vi "SIAM-7xRollingShutter.vi"() -> ()   [LabVIEW 2011]
uses:
  SIAM_command.ctl
panel:
  in  "Wob/µm":dbl=62.993226
  in  "Grid µm":dbl=29.0
  out "set Camera Exposure [µs]":dbl=743.175
  in  "PhaseImages":u16=7
  in  "GalvoX-Blanking":dbl
  in  "NoOfImages":u16=35
  out "µmShift":dbl=10.96096971726759 format="%#_8g"
  in  "Camera-Lines":u32=1082
  in  "Turn_ticks":u32=120
  in  "SM_ticks":u32=116
  in  "Trigger_ticks":u32=100
  in  "Mask_tpos":dbl=45853.0
  in  "LineTime-µs":dbl=27.525
  in  "RollingShutter height":u16=27
  in  "galvox/pixel":dbl=7.407
  in  "galvox-Line1080":dbl=-12220.0
  out "SIAMScript":T2(array[cluster])=[{"Delay 10µs"=50, "command"=1612709953, "P0"=0, "P1"=-269103235, "P2"=0, "P3"=0, "P4"=0, "P5-ticket"=0}, {"Delay 10µs"=0, "command"=1611661377, "P0"=0, "P1"=0, "P2"=0, "P3"=0, "P4"=0, "P5-ticket"=0}, {"Delay 10µs"=120, "command"=1612709921, "P0"=0, "P1"=0, "P2"=-2821727, "P3"=0, "P4"=0, "P5-ticket"=0}, {"Delay 10µs"=113, "command"=3506438145, "P0"=1, "P1"=1, "P2"=0, "P3"=0, "P4"=0, "P5-ticket"=0}, {"Delay 10µs"=100, "command"=3506438145, "P0"=1, "P1"=0, "P2"=0, "P3"=0, "P4"=0, "P5-ticket"=0}, {"Delay 10µs"=2856, "command"=1612709921, "P0"=0, "P1"=0, "P2"=0, "P3"=0, "P4"=0, "P5-ticket"=0}, {"Delay 10µs"=50, "command"=1612709953, "P0"=0, "P1"=-269103235, "P2"=0, "P3"=0, "P4"=0, "P5-ticket"=0}, {"Delay 10µs"=0, "command"=1611661377, "P0"=0, "P1"=45250435, "P2"=0, "P3"=0, "P4"=0, "P5-ticket"=0}, {"Delay 10µs"=120, "command"=1612709921, "P0"=0, "P1"=0, "P2"=-2821727, "P3"=0, "P4"=0, "P5-ticket"=0}, {"Delay 10µs"=113, "command"=3506438145, "P0"=1, "P1"=1, "P2"=0, "P3"=0, "P4"=0, "P5-ticket"=0}, {"Delay 10µs"=100, "command"=3506438145, "P0"=1, "P1"=0, "P2"=0, "P3"=0, "P4"=0, "P5-ticket"=0}, {"Delay 10µs"=2856, "command"=1612709921, "P0"=0, "P1"=0, "P2"=0, "P3"=0, "P4"=0, "P5-ticket"=0}, {"Delay 10µs"=50, "command"=1612709953, "P0"=0, "P1"=-269103235, "P2"=0, "P3"=0, "P4"=0, "P5-ticket"=0}, {"Delay 10µs"=0, "command"=1611661377, "P0"=0, "P1"=90500870, "P2"=0, "P3"=0, "P4"=0, "P5-ticket"=0}, {"Delay 10µs"=120, "command"=1612709921, "P0"=0, "P1"=0, "P2"=-2821727, "P3"=0, "P4"=0, "P5-ticket"=0}, {"Delay 10µs"=113, "command"=3506438145, "P0"=1, "P1"=1, "P2"=0, "P3"=0, "P4"=0, "P5-ticket"=0}, {"Delay 10µs"=100, "command"=3506438145, "P0"=1, "P1"=0, "P2"=0, "P3"=0, "P4"=0, "P5-ticket"=0}, {"Delay 10µs"=2856, "command"=1612709921, "P0"=0, "P1"=0, "P2"=0, "P3"=0, "P4"=0, "P5-ticket"=0}, {"Delay 10µs"=50, "command"=1612709953, "P0"=0, "P1"=-269103235, "P2"=0, "P3"=0, "P4"=0, "P5-ticket"=0}, {"Delay 10µs"=0, "command"=1611661377, "P0"=0, "P1"=135751305, "P2"=0, "P3"=0, "P4"=0, "P5-ticket"=0}, {"Delay 10µs"=120, "command"=1612709921, "P0"=0, "P1"=0, "P2"=-2821727, "P3"=0, "P4"=0, "P5-ticket"=0}, {"Delay 10µs"=113, "command"=3506438145, "P0"=1, "P1"=1, "P2"=0, "P3"=0, "P4"=0, "P5-ticket"=0}, {"Delay 10µs"=100, "command"=3506438145, "P0"=1, "P1"=0, "P2"=0, "P3"=0, "P4"=0, "P5-ticket"=0}, {"Delay 10µs"=2856, "command"=1612709921, "P0"=0, "P1"=0, "P2"=0, "P3"=0, "P4"=0, "P5-ticket"=0}, {"Delay 10µs"=50, "command"=1612709953, "P0"=0, "P1"=-269103235, "P2"=0, "P3"=0, "P4"=0, "P5-ticket"=0}, {"Delay 10µs"=0, "command"=1611661377, "P0"=0, "P1"=181001740, "P2"=0, "P3"=0, "P4"=0, "P5-ticket"=0}, {"Delay 10µs"=120, "command"=1612709921, "P0"=0, "P1"=0, "P2"=-2821727, "P3"=0, "P4"=0, "P5-ticket"=0}, {"Delay 10µs"=113, "command"=3506438145, "P0"=1, "P1"=1, "P2"=0, "P3"=0, "P4"=0, "P5-ticket"=0}, {"Delay 10µs"=100, "command"=3506438145, "P0"=1, "P1"=0, "P2"=0, "P3"=0, "P4"=0, "P5-ticket"=0}, {"Delay 10µs"=2856, "command"=1612709921, "P0"=0, "P1"=0, "P2"=0, "P3"=0, "P4"=0, "P5-ticket"=0}, {"Delay 10µs"=50, "command"=1612709953, "P0"=0, "P1"=-269103235, "P2"=0, "P3"=0, "P4"=0, "P5-ticket"=0}, {"Delay 10µs"=0, "command"=1611661377, "P0"=0, "P1"=226252175, "P2"=0, "P3"=0, "P4"=0, "P5-ticket"=0}, {"Delay 10µs"=120, "command"=1612709921, "P0"=0, "P1"=0, "P2"=-2821727, "P3"=0, "P4"=0, "P5-ticket"=0}, {"Delay 10µs"=113, "command"=3506438145, "P0"=1, "P1"=1, "P2"=0, "P3"=0, "P4"=0, "P5-ticket"=0}, {"Delay 10µs"=100, "command"=3506438145, "P0"=1, "P1"=0, "P2"=0, "P3"=0, "P4"=0, "P5-ticket"=0}, {"Delay 10µs"=2856, "command"=1612709921, "P0"=0, "P1"=0, "P2"=0, "P3"=0, "P4"=0, "P5-ticket"=0}, {"Delay 10µs"=50, "command"=1612709953, "P0"=0, "P1"=-269103235, "P2"=0, "P3"=0, "P4"=0, "P5-ticket"=0}, {"Delay 10µs"=0, "command"=1611661377, "P0"=0, "P1"=271502610, "P2"=0, "P3"=0, "P4"=0, "P5-ticket"=0}, {"Delay 10µs"=120, "command"=1612709921, "P0"=0, "P1"=0, "P2"=-2821727, "P3"=0, "P4"=0, "P5-ticket"=0}, {"Delay 10µs"=113, "command"=3506438145, "P0"=1, "P1"=1, "P2"=0, "P3"=0, "P4"=0, "P5-ticket"=0}, {"Delay 10µs"=100, "command"=3506438145, "P0"=1, "P1"=0, "P2"=0, "P3"=0, "P4"=0, "P5-ticket"=0}, {"Delay 10µs"=2856, "command"=1612709921, "P0"=0, "P1"=0, "P2"=0, "P3"=0, "P4"=0, "P5-ticket"=0}, {"Delay 10µs"=50, "command"=1612709953, "P0"=0, "P1"=-269103235, "P2"=0, "P3"=0, "P4"=0, "P5-ticket"=0}, {"Delay 10µs"=0, "command"=1611661377, "P0"=0, "P1"=316753045, "P2"=0, "P3"=0, "P4"=0, "P5-ticket"=0}, {"Delay 10µs"=120, "command"=1612709921, "P0"=0, "P1"=0, "P2"=-2821727, "P3"=0, "P4"=0, "P5-ticket"=0}, {"Delay 10µs"=113, "command"=3506438145, "P0"=1, "P1"=1, "P2"=0, "P3"=0, "P4"=0, "P5-ticket"=0}, {"Delay 10µs"=100, "command"=3506438145, "P0"=1, "P1"=0, "P2"=0, "P3"=0, "P4"=0, "P5-ticket"=0}, {"Delay 10µs"=2856, "command"=1612709921, "P0"=0, "P1"=0, "P2"=0, "P3"=0, "P4"=0, "P5-ticket"=0}, {"Delay 10µs"=50, "command"=1612709953, "P0"=0, "P1"=-269103235, "P2"=0, "P3"=0, "P4"=0, "P5-ticket"=0}, {"Delay 10µs"=0, "command"=1611661377, "P0"=0, "P1"=362003480, "P2"=0, "P3"=0, "P4"=0, "P5-ticket"=0}, {"Delay 10µs"=120, "command"=1612709921, "P0"=0, "P1"=0, "P2"=-2821727, "P3"=0, "P4"=0, "P5-ticket"=0}, {"Delay 10µs"=113, "command"=3506438145, "P0"=1, "P1"=1, "P2"=0, "P3"=0, "P4"=0, "P5-ticket"=0}, {"Delay 10µs"=100, "command"=3506438145, "P0"=1, "P1"=0, "P2"=0, "P3"=0, "P4"=0, "P5-ticket"=0}, {"Delay 10µs"=2856, "command"=1612709921, "P0"=0, "P1"=0, "P2"=0, "P3"=0, "P4"=0, "P5-ticket"=0}, {"Delay 10µs"=50, "command"=1612709953, "P0"=0, "P1"=-269103235, "P2"=0, "P3"=0, "P4"=0, "P5-ticket"=0}, {"Delay 10µs"=0, "command"=1611661377, "P0"=0, "P1"=407253915, "P2"=0, "P3"=0, "P4"=0, "P5-ticket"=0}, {"Delay 10µs"=120, "command"=1612709921, "P0"=0, "P1"=0, "P2"=-2821727, "P3"=0, "P4"=0, "P5-ticket"=0}, {"Delay 10µs"=113, "command"=3506438145, "P0"=1, "P1"=1, "P2"=0, "P3"=0, "P4"=0, "P5-ticket"=0}, {"Delay 10µs"=100, "command"=3506438145, "P0"=1, "P1"=0, "P2"=0, "P3"=0, "P4"=0, "P5-ticket"=0}, {"Delay 10µs"=2856, "command"=1612709921, "P0"=0, "P1"=0, "P2"=0, "P3"=0, "P4"=0, "P5-ticket"=0}, {"Delay 10µs"=50, "command"=1612709953, "P0"=0, "P1"=-269103235, "P2"=0, "P3"=0, "P4"=0, "P5-ticket"=0}, {"Delay 10µs"=0, "command"=1611661377, "P0"=0, "P1"=452504350, "P2"=0, "P3"=0, "P4"=0, "P5-ticket"=0}, {"Delay 10µs"=120, "command"=1612709921, "P0"=0, "P1"=0, "P2"=-2821727, "P3"=0, "P4"=0, "P5-ticket"=0}, {"Delay 10µs"=113, "command"=3506438145, "P0"=1, "P1"=1, "P2"=0, "P3"=0, "P4"=0, "P5-ticket"=0}, {"Delay 10µs"=100, "command"=3506438145, "P0"=1, "P1"=0, "P2"=0, "P3"=0, "P4"=0, "P5-ticket"=0}, {"Delay 10µs"=2856, "command"=1612709921, "P0"=0, "P1"=0, "P2"=0, "P3"=0, "P4"=0, "P5-ticket"=0}, {"Delay 10µs"=50, "command"=1612709953, "P0"=0, "P1"=-269103235, "P2"=0, "P3"=0, "P4"=0, "P5-ticket"=0}, {"Delay 10µs"=0, "command"=1611661377, "P0"=0, "P1"=497754785, "P2"=0, "P3"=0, "P4"=0, "P5-ticket"=0}, {"Delay 10µs"=120, "command"=1612709921, "P0"=0, "P1"=0, "P2"=-2821727, "P3"=0, "P4"=0, "P5-ticket"=0}, {"Delay 10µs"=113, "command"=3506438145, "P0"=1, "P1"=1, "P2"=0, "P3"=0, "P4"=0, "P5-ticket"=0}, {"Delay 10µs"=100, "command"=3506438145, "P0"=1, "P1"=0, "P2"=0, "P3"=0, "P4"=0, "P5-ticket"=0}, {"Delay 10µs"=2856, "command"=1612709921, "P0"=0, "P1"=0, "P2"=0, "P3"=0, "P4"=0, "P5-ticket"=0}, {"Delay 10µs"=50, "command"=1612709953, "P0"=0, "P1"=-269103235, "P2"=0, "P3"=0, "P4"=0, "P5-ticket"=0}, {"Delay 10µs"=0, "command"=1611661377, "P0"=0, "P1"=543005220, "P2"=0, "P3"=0, "P4"=0, "P5-ticket"=0}, {"Delay 10µs"=120, "command"=1612709921, "P0"=0, "P1"=0, "P2"=-2821727, "P3"=0, "P4"=0, "P5-ticket"=0}, {"Delay 10µs"=113, "command"=3506438145, "P0"=1, "P1"=1, "P2"=0, "P3"=0, "P4"=0, "P5-ticket"=0}, {"Delay 10µs"=100, "command"=3506438145, "P0"=1, "P1"=0, "P2"=0, "P3"=0, "P4"=0, "P5-ticket"=0}, {"Delay 10µs"=2856, "command"=1612709921, "P0"=0, "P1"=0, "P2"=0, "P3"=0, "P4"=0, "P5-ticket"=0}, {"Delay 10µs"=50, "command"=1612709953, "P0"=0, "P1"=-269103235, "P2"=0, "P3"=0, "P4"=0, "P5-ticket"=0}, {"Delay 10µs"=0, "command"=1611661377, "P0"=0, "P1"=588255655, "P2"=0, "P3"=0, "P4"=0, "P5-ticket"=0}, {"Delay 10µs"=120, "command"=1612709921, "P0"=0, "P1"=0, "P2"=-2821727, "P3"=0, "P4"=0, "P5-ticket"=0}, {"Delay 10µs"=113, "command"=3506438145, "P0"=1, "P1"=1, "P2"=0, "P3"=0, "P4"=0, "P5-ticket"=0}, {"Delay 10µs"=100, "command"=3506438145, "P0"=1, "P1"=0, "P2"=0, "P3"=0, "P4"=0, "P5-ticket"=0}, {"Delay 10µs"=2856, "command"=1612709921, "P0"=0, "P1"=0, "P2"=0, "P3"=0, "P4"=0, "P5-ticket"=0}, {"Delay 10µs"=50, "command"=1612709953, "P0"=0, "P1"=-269103235, "P2"=0, "P3"=0, "P4"=0, "P5-ticket"=0}, {"Delay 10µs"=0, "command"=1611661377, "P0"=0, "P1"=633506090, "P2"=0, "P3"=0, "P4"=0, "P5-ticket"=0}, {"Delay 10µs"=120, "command"=1612709921, "P0"=0, "P1"=0, "P2"=-2821727, "P3"=0, "P4"=0, "P5-ticket"=0}, {"Delay 10µs"=113, "command"=3506438145, "P0"=1, "P1"=1, "P2"=0, "P3"=0, "P4"=0, "P5-ticket"=0}, {"Delay 10µs"=100, "command"=3506438145, "P0"=1, "P1"=0, "P2"=0, "P3"=0, "P4"=0, "P5-ticket"=0}, {"Delay 10µs"=2856, "command"=1612709921, "P0"=0, "P1"=0, "P2"=0, "P3"=0, "P4"=0, "P5-ticket"=0}, {"Delay 10µs"=50, "command"=1612709953, "P0"=0, "P1"=-269103235, "P2"=0, "P3"=0, "P4"=0, "P5-ticket"=0}, {"Delay 10µs"=0, "command"=1611661377, "P0"=0, "P1"=678756525, "P2"=0, "P3"=0, "P4"=0, "P5-ticket"=0}, {"Delay 10µs"=120, "command"=1612709921, "P0"=0, "P1"=0, "P2"=-2821727, "P3"=0, "P4"=0, "P5-ticket"=0}, {"Delay 10µs"=113, "command"=3506438145, "P0"=1, "P1"=1, "P2"=0, "P3"=0, "P4"=0, "P5-ticket"=0}, {"Delay 10µs"=100, "command"=3506438145, "P0"=1, "P1"=0, "P2"=0, "P3"=0, "P4"=0, "P5-ticket"=0}, {"Delay 10µs"=2856, "command"=1612709921, "P0"=0, "P1"=0, "P2"=0, "P3"=0, "P4"=0, "P5-ticket"=0}, {"Delay 10µs"=50, "command"=1612709953, "P0"=0, "P1"=-269103235, "P2"=0, "P3"=0, "P4"=0, "P5-ticket"=0}, {"Delay 10µs"=0, "command"=1611661377, "P0"=0, "P1"=724006960, "P2"=0, "P3"=0, "P4"=0, "P5-ticket"=0}, {"Delay 10µs"=120, "command"=1612709921, "P0"=0, "P1"=0, "P2"=-2821727, "P3"=0, "P4"=0, "P5-ticket"=0}, {"Delay 10µs"=113, "command"=3506438145, "P0"=1, "P1"=1, "P2"=0, "P3"=0, "P4"=0, "P5-ticket"=0}, {"Delay 10µs"=100, "command"=3506438145, "P0"=1, "P1"=0, "P2"=0, "P3"=0, "P4"=0, "P5-ticket"=0}, {"Delay 10µs"=2856, "command"=1612709921, "P0"=0, "P1"=0, "P2"=0, "P3"=0, "P4"=0, "P5-ticket"=0}, {"Delay 10µs"=50, "command"=1612709953, "P0"=0, "P1"=-269103235, "P2"=0, "P3"=0, "P4"=0, "P5-ticket"=0}, {"Delay 10µs"=0, "command"=1611661377, "P0"=0, "P1"=769257395, "P2"=0, "P3"=0, "P4"=0, "P5-ticket"=0}, {"Delay 10µs"=120, "command"=1612709921, "P0"=0, "P1"=0, "P2"=-2821727, "P3"=0, "P4"=0, "P5-ticket"=0}, {"Delay 10µs"=113, "command"=3506438145, "P0"=1, "P1"=1, "P2"=0, "P3"=0, "P4"=0, "P5-ticket"=0}, {"Delay 10µs"=100, "command"=3506438145, "P0"=1, "P1"=0, "P2"=0, "P3"=0, "P4"=0, "P5-ticket"=0}, {"Delay 10µs"=2856, "command"=1612709921, "P0"=0, "P1"=0, "P2"=0, "P3"=0, "P4"=0, "P5-ticket"=0}, {"Delay 10µs"=50, "command"=1612709953, "P0"=0, "P1"=-269103235, "P2"=0, "P3"=0, "P4"=0, "P5-ticket"=0}, {"Delay 10µs"=0, "command"=1611661377, "P0"=0, "P1"=814507830, "P2"=0, "P3"=0, "P4"=0, "P5-ticket"=0}, {"Delay 10µs"=120, "command"=1612709921, "P0"=0, "P1"=0, "P2"=-2821727, "P3"=0, "P4"=0, "P5-ticket"=0}, {"Delay 10µs"=113, "command"=3506438145, "P0"=1, "P1"=1, "P2"=0, "P3"=0, "P4"=0, "P5-ticket"=0}, {"Delay 10µs"=100, "command"=3506438145, "P0"=1, "P1"=0, "P2"=0, "P3"=0, "P4"=0, "P5-ticket"=0}, {"Delay 10µs"=2856, "command"=1612709921, "P0"=0, "P1"=0, "P2"=0, "P3"=0, "P4"=0, "P5-ticket"=0}, {"Delay 10µs"=50, "command"=1612709953, "P0"=0, "P1"=-269103235, "P2"=0, "P3"=0, "P4"=0, "P5-ticket"=0}, {"Delay 10µs"=0, "command"=1611661377, "P0"=0, "P1"=859758265, "P2"=0, "P3"=0, "P4"=0, "P5-ticket"=0}, {"Delay 10µs"=120, "command"=1612709921, "P0"=0, "P1"=0, "P2"=-2821727, "P3"=0, "P4"=0, "P5-ticket"=0}, {"Delay 10µs"=113, "command"=3506438145, "P0"=1, "P1"=1, "P2"=0, "P3"=0, "P4"=0, "P5-ticket"=0}, {"Delay 10µs"=100, "command"=3506438145, "P0"=1, "P1"=0, "P2"=0, "P3"=0, "P4"=0, "P5-ticket"=0}, {"Delay 10µs"=2856, "command"=1612709921, "P0"=0, "P1"=0, "P2"=0, "P3"=0, "P4"=0, "P5-ticket"=0}, {"Delay 10µs"=50, "command"=1612709953, "P0"=0, "P1"=-269103235, "P2"=0, "P3"=0, "P4"=0, "P5-ticket"=0}, {"Delay 10µs"=0, "command"=1611661377, "P0"=0, "P1"=905008700, "P2"=0, "P3"=0, "P4"=0, "P5-ticket"=0}, {"Delay 10µs"=120, "command"=1612709921, "P0"=0, "P1"=0, "P2"=-2821727, "P3"=0, "P4"=0, "P5-ticket"=0}, {"Delay 10µs"=113, "command"=3506438145, "P0"=1, "P1"=1, "P2"=0, "P3"=0, "P4"=0, "P5-ticket"=0}, {"Delay 10µs"=100, "command"=3506438145, "P0"=1, "P1"=0, "P2"=0, "P3"=0, "P4"=0, "P5-ticket"=0}, {"Delay 10µs"=2856, "command"=1612709921, "P0"=0, "P1"=0, "P2"=0, "P3"=0, "P4"=0, "P5-ticket"=0}, {"Delay 10µs"=50, "command"=1612709953, "P0"=0, "P1"=-269103235, "P2"=0, "P3"=0, "P4"=0, "P5-ticket"=0}, {"Delay 10µs"=0, "command"=1611661377, "P0"=0, "P1"=950259135, "P2"=0, "P3"=0, "P4"=0, "P5-ticket"=0}, {"Delay 10µs"=120, "command"=1612709921, "P0"=0, "P1"=0, "P2"=-2821727, "P3"=0, "P4"=0, "P5-ticket"=0}, {"Delay 10µs"=113, "command"=3506438145, "P0"=1, "P1"=1, "P2"=0, "P3"=0, "P4"=0, "P5-ticket"=0}, {"Delay 10µs"=100, "command"=3506438145, "P0"=1, "P1"=0, "P2"=0, "P3"=0, "P4"=0, "P5-ticket"=0}, {"Delay 10µs"=2856, "command"=1612709921, "P0"=0, "P1"=0, "P2"=0, "P3"=0, "P4"=0, "P5-ticket"=0}, {"Delay 10µs"=50, "command"=1612709953, "P0"=0, "P1"=-269103235, "P2"=0, "P3"=0, "P4"=0, "P5-ticket"=0}, {"Delay 10µs"=0, "command"=1611661377, "P0"=0, "P1"=995509570, "P2"=0, "P3"=0, "P4"=0, "P5-ticket"=0}, {"Delay 10µs"=120, "command"=1612709921, "P0"=0, "P1"=0, "P2"=-2821727, "P3"=0, "P4"=0, "P5-ticket"=0}, {"Delay 10µs"=113, "command"=3506438145, "P0"=1, "P1"=1, "P2"=0, "P3"=0, "P4"=0, "P5-ticket"=0}, {"Delay 10µs"=100, "command"=3506438145, "P0"=1, "P1"=0, "P2"=0, "P3"=0, "P4"=0, "P5-ticket"=0}, {"Delay 10µs"=2856, "command"=1612709921, "P0"=0, "P1"=0, "P2"=0, "P3"=0, "P4"=0, "P5-ticket"=0}, {"Delay 10µs"=50, "command"=1612709953, "P0"=0, "P1"=-269103235, "P2"=0, "P3"=0, "P4"=0, "P5-ticket"=0}, {"Delay 10µs"=0, "command"=1611661377, "P0"=0, "P1"=1040760005, "P2"=0, "P3"=0, "P4"=0, "P5-ticket"=0}, {"Delay 10µs"=120, "command"=1612709921, "P0"=0, "P1"=0, "P2"=-2821727, "P3"=0, "P4"=0, "P5-ticket"=0}, {"Delay 10µs"=113, "command"=3506438145, "P0"=1, "P1"=1, "P2"=0, "P3"=0, "P4"=0, "P5-ticket"=0}, {"Delay 10µs"=100, "command"=3506438145, "P0"=1, "P1"=0, "P2"=0, "P3"=0, "P4"=0, "P5-ticket"=0}, {"Delay 10µs"=2856, "command"=1612709921, "P0"=0, "P1"=0, "P2"=0, "P3"=0, "P4"=0, "P5-ticket"=0}, {"Delay 10µs"=50, "command"=1612709953, "P0"=0, "P1"=-269103235, "P2"=0, "P3"=0, "P4"=0, "P5-ticket"=0}, {"Delay 10µs"=0, "command"=1611661377, "P0"=0, "P1"=1086010440, "P2"=0, "P3"=0, "P4"=0, "P5-ticket"=0}, {"Delay 10µs"=120, "command"=1612709921, "P0"=0, "P1"=0, "P2"=-2821727, "P3"=0, "P4"=0, "P5-ticket"=0}, {"Delay 10µs"=113, "command"=3506438145, "P0"=1, "P1"=1, "P2"=0, "P3"=0, "P4"=0, "P5-ticket"=0}, {"Delay 10µs"=100, "command"=3506438145, "P0"=1, "P1"=0, "P2"=0, "P3"=0, "P4"=0, "P5-ticket"=0}, {"Delay 10µs"=2856, "command"=1612709921, "P0"=0, "P1"=0, "P2"=0, "P3"=0, "P4"=0, "P5-ticket"=0}, {"Delay 10µs"=50, "command"=1612709953, "P0"=0, "P1"=0, "P2"=0, "P3"=0, "P4"=0, "P5-ticket"=0}, {"Delay 10µs"=10, "command"=4027518991, "P0"=0, "P1"=0, "P2"=0, "P3"=0, "P4"=0, "P5-ticket"=12345}] {"command" format="%x" items=["read_x-Motor_status_ticket"=17305600, "init_x-Motor"=17760263, "read_x-Motor_absolute_ticket"=16781312, "move_x-Motor_absolute"=16777217, "move_x-Motor_relative"=16842753, "read_y-Motor_status_ticket"=18354176, "init_y-Motor"=18808839, "read_y-Motor_absolute_ticket"=17829888, "move_y-Motor_absolute"=17825793, "move_y-Motor_relative"=17891329, "read_z-Motor_status_ticket"=19402752, "init_z-Motor"=19857415, "stop_z-Motor"=19857423, "start_z-Motor"=19857422, "read_z-Motor_absolute_ticket"=18878464, "move_z-Motor_absolute"=18874369, "move_z-Motor_relative"=18939905, "end_no_ticket"=4027514895, "end_ticket"=4027518991, "IO-read_bank0"=3489665024, "IO-write_bank0"=3489660929, "IO-read_bank1"=3506442240, "IO-write_bank1"=3506438145, "Analog-write_DA0-0"=2684354561, "Analog-write_DA0-1"=2685403137, "Analog-write_DA0-2"=2686451713, "Analog-write_DA0-3"=2687500289, "Analog-write_DA0-4"=2688548865, "Analog-write_DA0-5"=2689597441, "Analog-write_DA0-6"=2690646017, "Analog-write_DA0-7"=2691694593, "Analog-write_DA1-0"=2701131777, "Analog-write_DA1-1"=2702180353, "Analog-write_DA1-2"=2703228929, "Analog-write_DA1-3"=2704277505, "Analog-write_DA1-4"=2705326081, "Analog-write_DA1-5"=2706374657, "Analog-write_DA1-6"=2707423233, "Analog-write_DA1-7"=2708471809, "Analog-read_AD0-0"=2818576384, "Analog-read-store_AD0-0"=2818572290, "IO-delay_bank0"=3489923073, "IO-delay_bank0_fromVar"=3489923075, "read_cam_clock"=3289124864, "store_cam_clock"=3289120770, "read_cam_phase"=3289190400, "set_cam_deadtime"=3288989697, "set_cam_10uscycles"=3289055233, "set_cam_10uscycles_fromVariable"=3289055235, "calc_cam"=3289317386, "store_cam_Var"=3289251842, "math_addToVariable"=4060086278, "readVar"=4060090368, "writeVar"=4060086273, "copyVar"=4060086276, "decrement_branchRel_if_equal"=4043374945, "decrement_branchRel_if_greaterequal"=4043375201, "decrement_branchRel_if_greaterequal_withTicket"=4043379297, "decrement_branchRel_if_smaller"=4043375457, "increment_branchRel_if_smaller"=4043375473, "set_x-Galvo"=1612710129, "set_y-Galvo"=1613758705, "set_z-Fokus"=1614807281, "set_x-Galvo_position-only"=1612709953, "set_y-Galvo_position-only"=1613758529, "set_z-Fokus_position-only"=1614807105, "set_x-Galvo_position-only_ticket"=1612714049, "set_y-Galvo_position-only_ticket"=1613762625, "set_z-Fokus_position-only_ticket"=1614811201, "set_x-Galvo_speed-only"=1612709921, "set_y-Galvo_speed-only"=1613758497, "set_z-Fokus_speed-only"=1614807073, "read_x-Galvo_ticket"=1612714048, "read_y-Galvo_ticket"=1613762624, "read_z-Focus_ticket"=1614811200, "x-Galvo_pos_fromVar"=1612709955, "y-Galvo_pos_fromVar"=1613758531, "z-Focus_pos_fromVar"=1614807107]}
  # "jetzt x-wob orthogonal"
  # "29er/7=45250435"
  # "22/25,5/29"
  # "12,75+-0,02"
  # "12,75: 25,5\n14,4956: 29er"
  # "29 full wobbel=4833,267908cnt\n/sqrt(7) =1826,803557\n/29=62,993226 wob/µm"
  # "Zum einstellnen der 19.1°\ngemessen +0,0068°/step, 0bei 291,6°\ntheorie +0,00703°/step"
  # "tilcal 1\nspeed 50\nidmax"
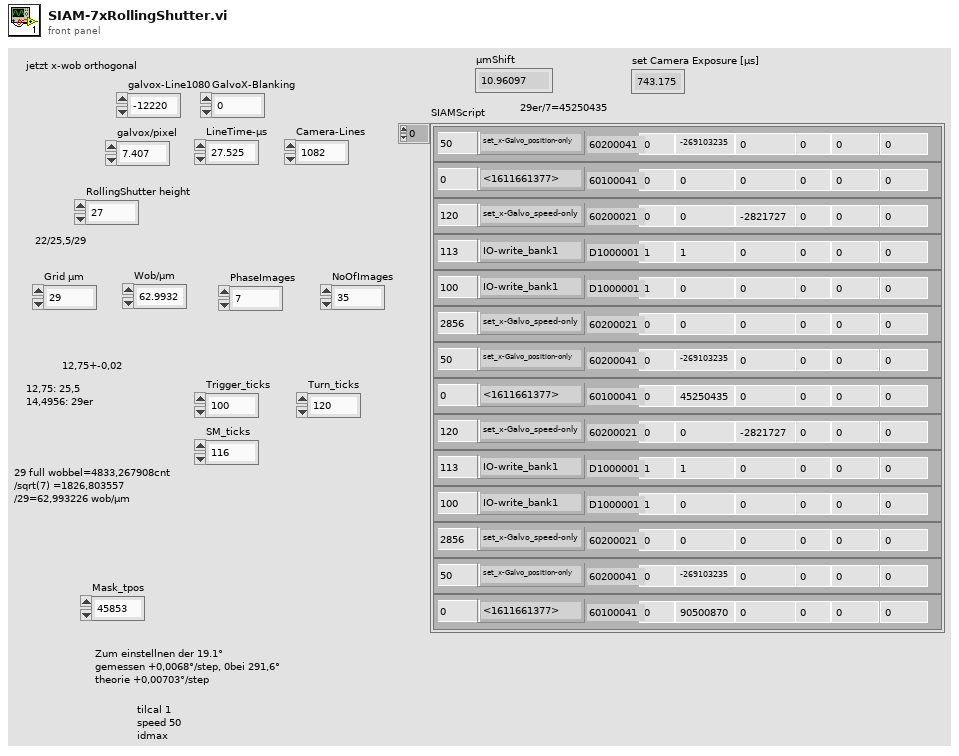
[diagram p1: front panel]
types:
  T1 = typedef "SIAM_command.ctl" = u32
  T2 = cluster{"Delay 10µs":u32, "command":T1, "P0":i32, "P1":i32, "P2":i32, "P3":i32, "P4":i32, "P5-ticket":i32}[]
  T3 = enum8{"Ch0", "Ch1", "x-Galvo", "y-Galvo", "z-Focus"}
  T4 = cluster{"Delay 10µs":u32, "command":T1, "P0":i32, "P1":i32, "P2":i32, "P3":i32, "P4":i32, "P5-ticket":i32}
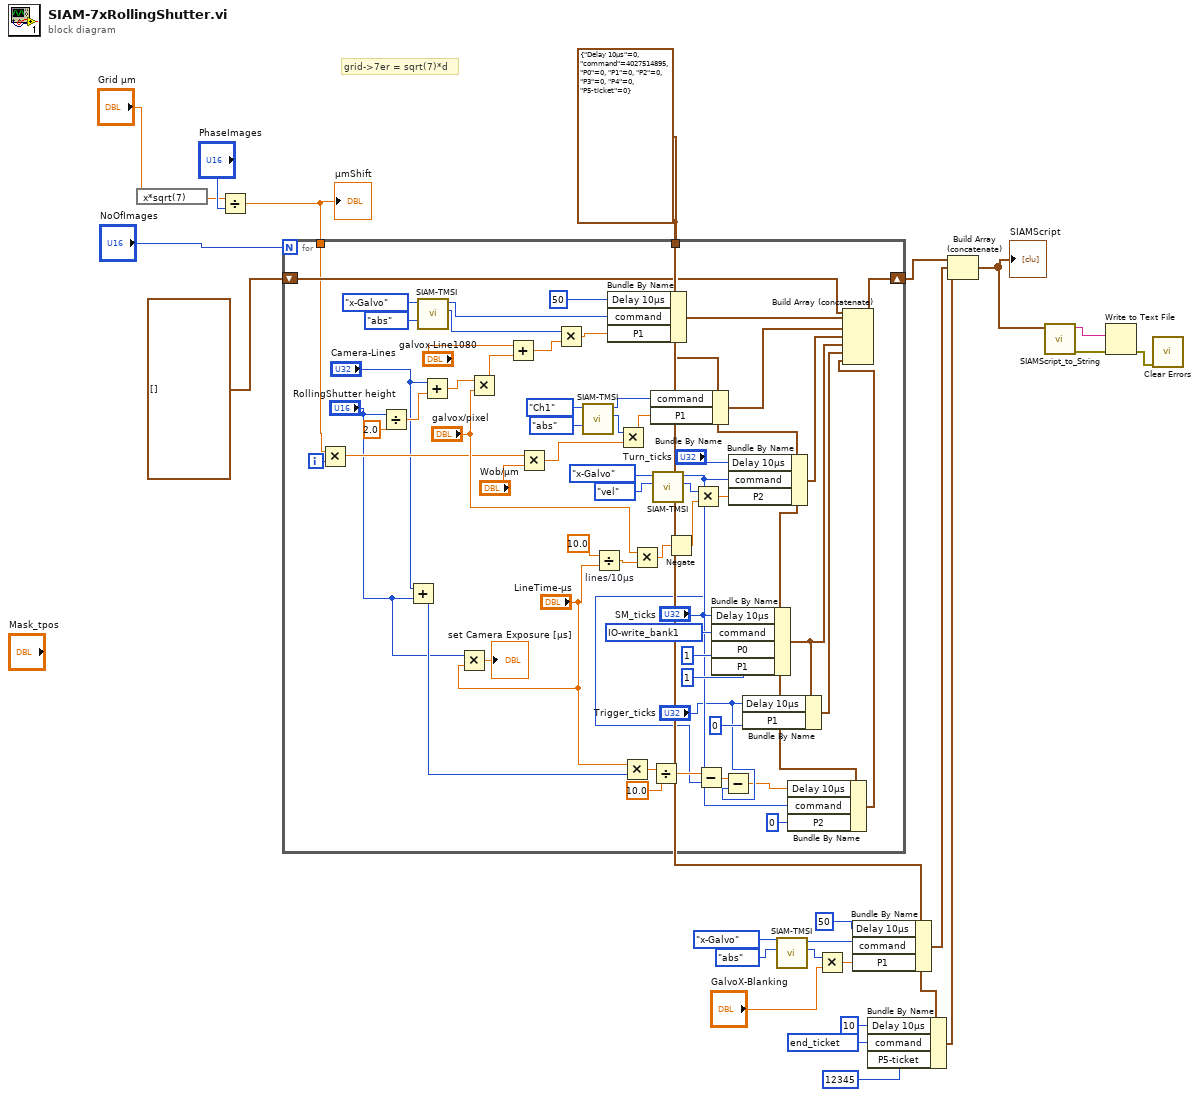
[diagram p0: block diagram]
diagram:
  w11 = T1 4027518991 items=["read_x-Motor_status_ticket"=17305600, "init_x-Motor"=17760263, "read_x-Motor_absolute_ticket"=16781312, "move_x-Motor_absolute"=16777217, "move_x-Motor_relative"=16842753, "read_y-Motor_status_ticket"=18354176, "init_y-Motor"=18808839, "read_y-Motor_absolute_ticket"=17829888, "move_y-Motor_absolute"=17825793, "move_y-Motor_relative"=17891329, "read_z-Motor_status_ticket"=19402752, "init_z-Motor"=19857415, "stop_z-Motor"=19857423, "start_z-Motor"=19857422, "read_z-Motor_absolute_ticket"=18878464, "move_z-Motor_absolute"=18874369, "move_z-Motor_relative"=18939905, "end_no_ticket"=4027514895, "end_ticket"=4027518991, "IO-read_bank0"=3489665024, "IO-write_bank0"=3489660929, "IO-read_bank1"=3506442240, "IO-write_bank1"=3506438145, "IO-delay_bank0"=3489923073, "IO-delay_bank0_fromVar"=3489923075, "read_cam_clock"=3289124864, "store_cam_clock"=3289120770, "read_cam_phase"=3289190400, "set_cam_deadtime"=3288989697, "set_cam_10uscycles"=3289055233, "set_cam_10uscycles_fromVariable"=3289055235, "calc_cam"=3289317386, "store_cam_Var"=3289251842, "math_addToVariable"=4060086278, "readVar"=4060090368, "writeVar"=4060086273, "copyVar"=4060086276, "decrement_branchRel_if_equal"=4043374945, "decrement_branchRel_if_greaterequal"=4043375201, "decrement_branchRel_if_greaterequal_withTicket"=4043379297, "decrement_branchRel_if_smaller"=4043375457, "increment_branchRel_if_smaller"=4043375473, "set_x-Galvo"=1612710129, "set_y-Galvo"=1613758705, "set_z-Fokus"=1614807281, "set_x-Galvo_position-only"=1612709953, "set_y-Galvo_position-only"=1613758529, "set_z-Fokus_position-only"=1614807105, "set_x-Galvo_position-only_ticket"=1612714049, "set_y-Galvo_position-only_ticket"=1613762625, "set_z-Fokus_position-only_ticket"=1614811201, "read_x-Galvo_ticket"=1612714048, "read_y-Galvo_ticket"=1613762624, "read_z-Focus_ticket"=1614811200, "x-Galvo_pos_fromVar"=1612709955, "y-Galvo_pos_fromVar"=1613758531, "z-Focus_pos_fromVar"=1614807107] ("command")
  w12 = T4 {"Delay 10µs"=0, "command"=4027514895, "P0"=0, "P1"=0, "P2"=0, "P3"=0, "P4"=0, "P5-ticket"=0} ("Cluster")
  # "grid->7er = sqrt(7)*d"
  n1 = expression code="x*sqrt(7)"("Grid µm") -> (w1:dbl)
  n2 = Divide(x=w1, y="PhaseImages") -> (x/y=w21:dbl)
  "µmShift" <- w21
  n3 = for {
    N: "NoOfImages" -> [_]
    tunnel: w21 -> [w35]
    tunnel: w12 -> [w50]
    shift-right: [w39] -> w23
    shift-left: T2 [] -> [w38]
    i -> [w36]
    w56 = T1 3506438145 items=["read_x-Motor_status_ticket"=17305600, "init_x-Motor"=17760263, "read_x-Motor_absolute_ticket"=16781312, "move_x-Motor_absolute"=16777217, "move_x-Motor_relative"=16842753, "read_y-Motor_status_ticket"=18354176, "init_y-Motor"=18808839, "read_y-Motor_absolute_ticket"=17829888, "move_y-Motor_absolute"=17825793, "move_y-Motor_relative"=17891329, "read_z-Motor_status_ticket"=19402752, "init_z-Motor"=19857415, "stop_z-Motor"=19857423, "start_z-Motor"=19857422, "read_z-Motor_absolute_ticket"=18878464, "move_z-Motor_absolute"=18874369, "move_z-Motor_relative"=18939905, "end_no_ticket"=4027514895, "end_ticket"=4027518991, "IO-read_bank0"=3489665024, "IO-write_bank0"=3489660929, "IO-read_bank1"=3506442240, "IO-write_bank1"=3506438145, "IO-delay_bank0"=3489923073, "IO-delay_bank0_fromVar"=3489923075, "read_cam_clock"=3289124864, "store_cam_clock"=3289120770, "read_cam_phase"=3289190400, "set_cam_deadtime"=3288989697, "set_cam_10uscycles"=3289055233, "set_cam_10uscycles_fromVariable"=3289055235, "calc_cam"=3289317386, "store_cam_Var"=3289251842, "math_addToVariable"=4060086278, "readVar"=4060090368, "writeVar"=4060086273, "copyVar"=4060086276, "decrement_branchRel_if_equal"=4043374945, "decrement_branchRel_if_greaterequal"=4043375201, "decrement_branchRel_if_greaterequal_withTicket"=4043379297, "decrement_branchRel_if_smaller"=4043375457, "increment_branchRel_if_smaller"=4043375473, "set_x-Galvo"=1612710129, "set_y-Galvo"=1613758705, "set_z-Fokus"=1614807281, "set_x-Galvo_position-only"=1612709953, "set_y-Galvo_position-only"=1613758529, "set_z-Fokus_position-only"=1614807105, "set_x-Galvo_position-only_ticket"=1612714049, "set_y-Galvo_position-only_ticket"=1613762625, "set_z-Fokus_position-only_ticket"=1614811201, "read_x-Galvo_ticket"=1612714048, "read_y-Galvo_ticket"=1613762624, "read_z-Focus_ticket"=1614811200, "x-Galvo_pos_fromVar"=1612709955, "y-Galvo_pos_fromVar"=1613758531, "z-Focus_pos_fromVar"=1614807107] ("command")
    n4 = Multiply(x=w35, y=w36) -> (x*y=w34:dbl)
    n5 = Divide(x="RollingShutter height", y=2.0) -> (x/y=w79:dbl)
    n6 = Add(x="Camera-Lines", y="RollingShutter height") -> (x+y=w31:u32)
    n7 = call "SIAM-TMSI.vi"("Type"=enum8{"acc", "vel", "abs", "offset"}."abs", "Motor"=T3."x-Galvo") -> ("Resolution-Factor"=w75:i32, "command"=w81:T1)  [unwired: 6 in, 2 out]
    n8 = Add(x="Camera-Lines", y=w79) -> (x+y=w26:dbl)
    n9 = Multiply(x="RollingShutter height", y="LineTime-µs") -> (x*y=→"set Camera Exposure [µs]":dbl)
    n10 = Multiply(x=w26, y="galvox/pixel") -> (x*y=w78:dbl)
    n11 = Add(x="galvox-Line1080", y=w78) -> (x+y=w76:dbl)
    n12 = Multiply(x=w34, y="Wob/µm") -> (x*y=w67:dbl)
    n13 = Multiply(x=w75, y=w76) -> (x*y=w74:dbl)
    n14 = call "SIAM-TMSI.vi"("Type"=enum8{"acc", "vel", "abs", "offset"}."abs", "Motor"=T3."Ch1") -> ("Resolution-Factor"=w68:i32, "command"=w69:T1)  [unwired: 6 in, 2 out]
    n15 = Divide "lines/10µs"(x=10.0 ("y"), y="LineTime-µs") -> (x/y=w59:dbl)
    n16 = Bundle By Name(cluster=w50, "Delay 10µs"=u32 50, "command"=w81, "P1"=w74) -> (w73:T4)
    n17 = Multiply(x=w68, y=w67) -> (x*y=w66:dbl)
    n18 = Multiply(x="LineTime-µs", y=w31) -> (x*y=w47:dbl)
    n19 = Multiply(x="galvox/pixel", y=w59) -> (x*y=w57:dbl)
    n20 = Bundle By Name(cluster=w50, "command"=w69, "P1"=w66) -> (w72:T4)
    n21 = Divide(x=w47, y=10.0) -> (x/y=w45:dbl)
    n22 = call "SIAM-TMSI.vi"("Type"=enum8{"acc", "vel", "abs", "offset"}."vel", "Motor"=T3."x-Galvo") -> ("Resolution-Factor"=w61:i32, "command"=w48:T1)  [unwired: 6 in, 2 out]
    n23 = Negate(x=w57) -> (-x=w37:dbl)
    n24 = Multiply(x=w61, y=w37) -> (x*y=w62:dbl)
    n25 = Subtract(x=w45, y="SM_ticks") -> (x-y=w43:dbl)
    n26 = Bundle By Name(cluster=w50, "Delay 10µs"="SM_ticks", "command"=w56, "P0"=1, "P1"=1) -> (w53:T4)
    n27 = Subtract(x=w43, y="Trigger_ticks") -> (x-y=w41:dbl)
    n28 = Bundle By Name(cluster=w50, "Delay 10µs"="Turn_ticks", "command"=w48, "P2"=w62) -> (w63:T4)
    n29 = Bundle By Name(cluster=w53, "Delay 10µs"="Trigger_ticks", "P1"=0) -> (w51:T4)
    n30 = Bundle By Name(cluster=w50, "Delay 10µs"=w41, "command"=w48, "P2"=0) -> (w40:T4)
    n31 = Build Array (concatenate)(w38, w73, w72, w63, w53, w51, w40) -> (w39:T2)
  }
  n32 = call "SIAM-TMSI.vi"("Type"=enum8{"acc", "vel", "abs", "offset"}."abs", "Motor"=T3."x-Galvo") -> ("Resolution-Factor"=w17:i32, "command"=w16:T1)  [unwired: 6 in, 2 out]
  n33 = Multiply(x=w17, y="GalvoX-Blanking") -> (x*y=w18:dbl)
  n34 = Bundle By Name(cluster=w12, "Delay 10µs"=u32 50, "command"=w16, "P1"=w18) -> (w13:T4)
  n35 = Bundle By Name(cluster=w12, "Delay 10µs"=u32 10, "command"=w11, "P5-ticket"=12345) -> (w9:T4)
  n36 = Build Array (concatenate)(w23, w13, w9) -> (w7:T2)
  "SIAMScript" <- w7
  n37 = call "SIAMScript_to_String.vi"("Script"=w7) -> ("error out"=w5:errorcluster, "String"=w6:string)  [unwired: 9 in]
  n38 = Write to Text File(text=w6, error in=w5) -> (error out=w4:errorcluster)  [unwired: 2 in, 2 out]
  n39 = call <vilib>:"Clear Errors.vi"("error in (no error)"=w4) -> ()  [unwired: 6 in, 1 out]
